vi "QMH_Demo_1.vi"(11 "Sender":string="Demo_1") -> ()   [LabVIEW 2014]
panel:
  in  "Receiver":string="Demo"
  out "Receive data":string
  in  "Send data":string
  in  "STOP":bool
  in  "send":bool
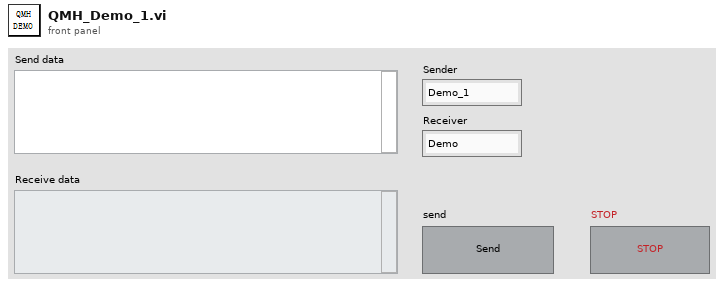
[diagram p1: front panel]
types:
  T1 = cluster{"Communication message":cluster{"Sender":string, "receiver":string, "message":string, "data":variant}, "Receive data":string}
  T2 = cluster{"Sender":string, "receiver":string, "message":string, "data":variant}
  T3 = enum32{"invalid app kind", "Development System", "Run Time System", "Student Edition", "Embedded LabVIEW", "Evaluation", "Custom"}
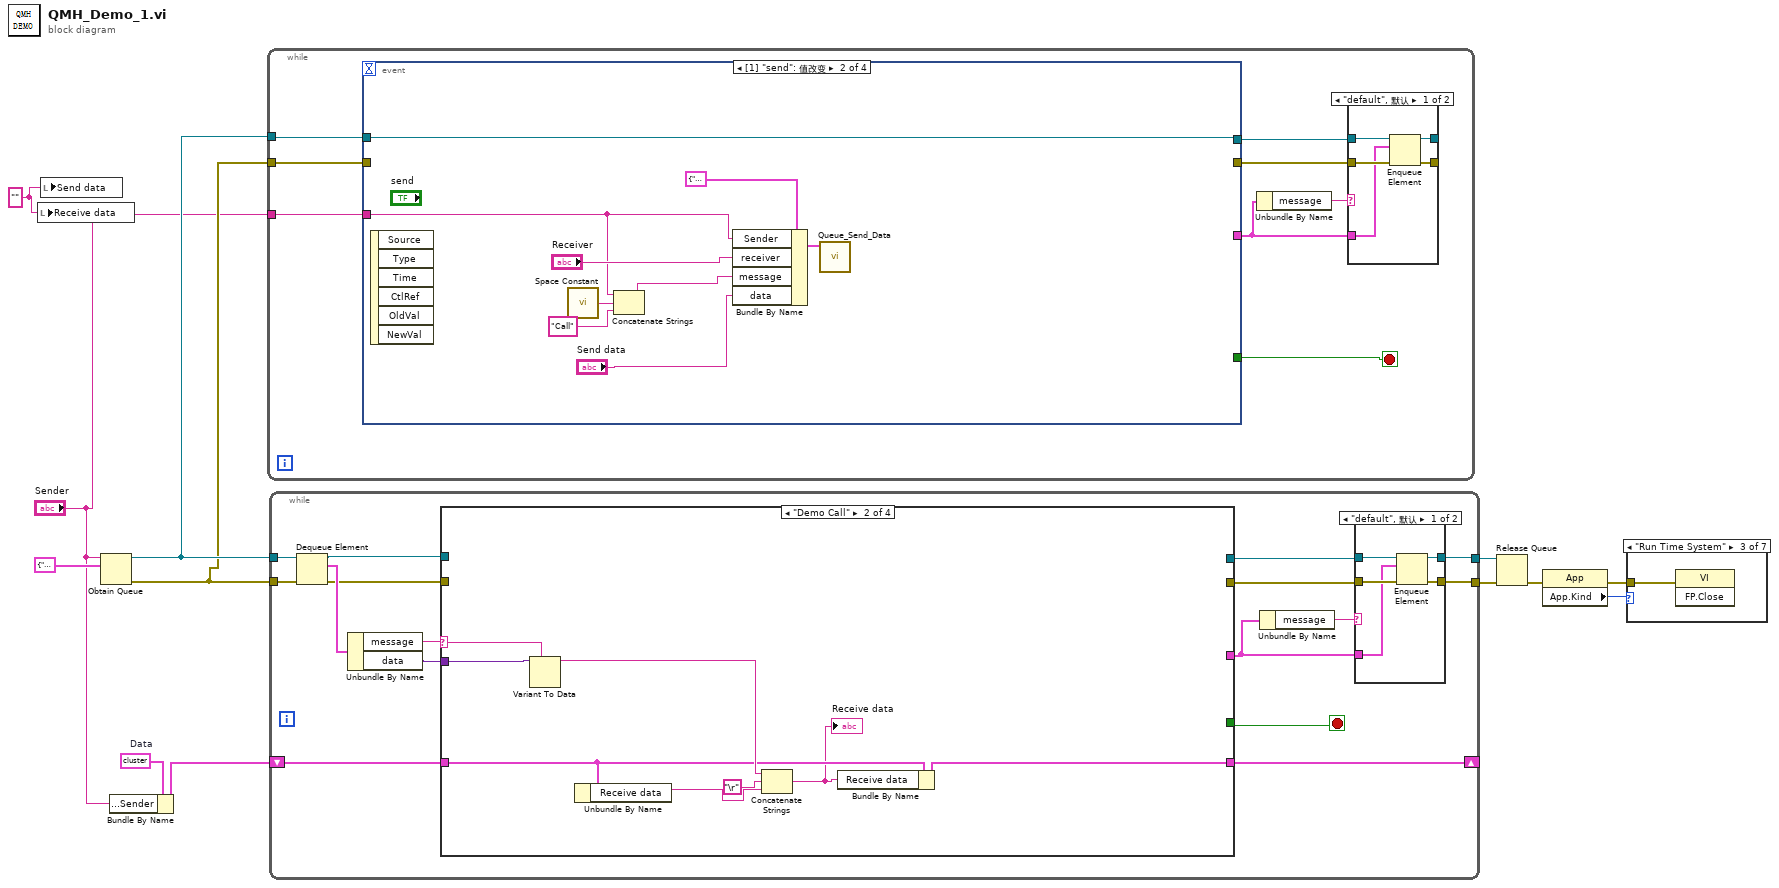
[diagram p0: block diagram]
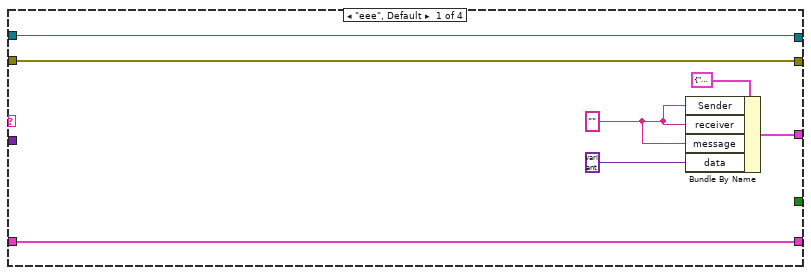
[diagram p9: hidden frame]
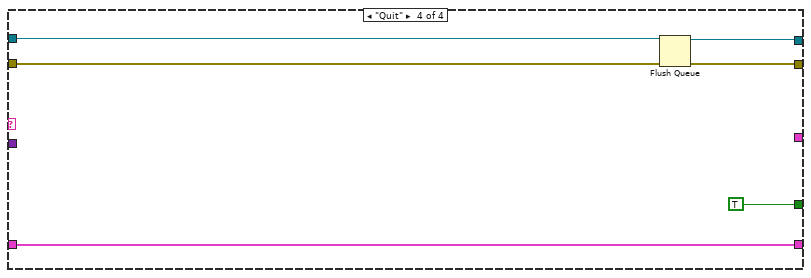
[diagram p11: hidden frame]
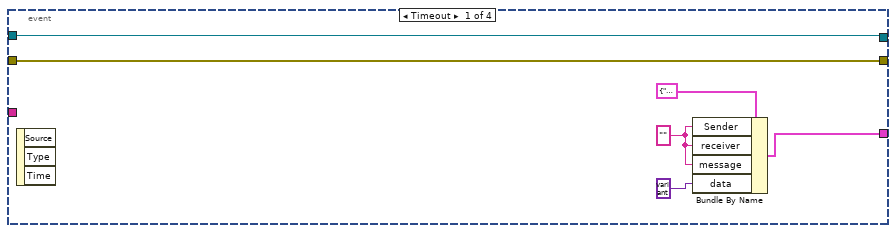
[diagram p13: hidden frame]
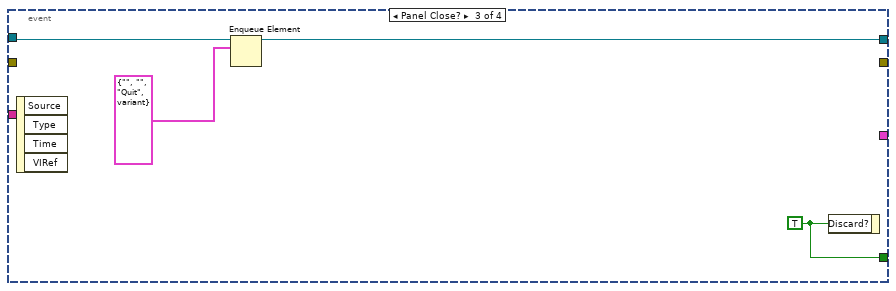
[diagram p14: hidden frame]
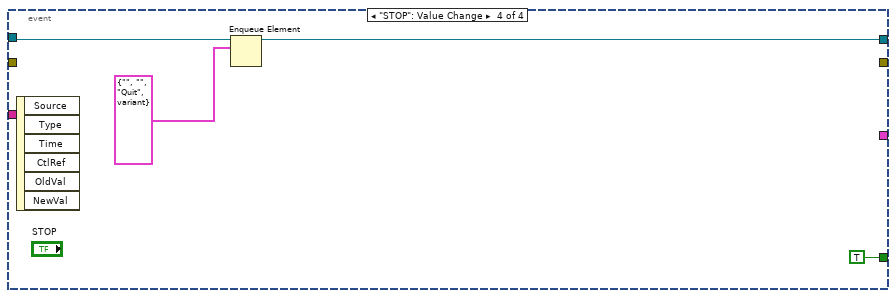
[diagram p15: hidden frame]
diagram:
  w1 = "" ("message")
  w4 = T1 {"Communication message"={"Sender"="", "receiver"="", "message"="", "data"=variant}, "Receive data"=""}  # Data
  n1 = local write "Receive data"(w1) -> ()
  n2 = local write "Send data"(w1) -> ()
  n3 = Obtain Queue(name (unnamed)="Sender", element data type=T2 {"Sender"="", "receiver"="", "message"="", "data"=variant} ("Communication message")) -> (queue out=w12:refnum<queue>, error out=w5:errorcluster)  [unwired: 3 in, 1 out]
  n4 = Bundle By Name(cluster=w4, "Communication message.Sender"="Sender") -> (w3:T1)
  n5 = while {
    tunnel: w12 -> [w19]
    tunnel: w5 -> [w17]
    tunnel: "Sender" -> [w13]
    stop <- w20 stop-if-true
    n6 = event shown="[1] \"send\": 值改变" {
      selector: _ -> [_ _ _ _]
      dyn-events: _ -> [_ _ _ _]
      timeout: _ -> [_ _ _ _]
      tunnel: [_ _ w46 TRUE ("放弃？")] -> w20
      tunnel: w19 -> [w30 w42 w45 w49]
      tunnel: [w30 w42 w43 w47] -> w18
      tunnel: [w32 _ _ _] -> w15
      tunnel: [w29 _ _ _] -> w16
      tunnel: w17 -> [w29 _ _ _]
      tunnel: w13 -> [_ w36 _ _]
      event Timeout {
        w28 = ""
        n7 = event-data() -> ()  [unwired: 1 in, 3 out]
        n8 = Bundle By Name(cluster=T2 {"Sender"="", "receiver"="", "message"="", "data"=variant} ("Communication message"), "Sender"=w28, "receiver"=w28, "message"=w28, "data"=variant) -> (w32:T2)
      }
      event "send": Value Change {
        n9 = event-data() -> ()  [unwired: 1 in, 6 out]
        n10 = call <vilib>:"Space Constant.vi"() -> ("String"=w35:string)
        n11 = Concatenate Strings(w36, w35, "Call" ("message")) -> (w37:string)
        n12 = Bundle By Name(cluster=T2 {"Sender"="", "receiver"="", "message"="", "data"=variant} ("Communication message"), "Sender"=w36, "receiver"="Receiver", "message"=w37, "data"="Send data") -> (w40:T2)
        n13 = call "Queue_Send_Data.vi"("Communication message"=w40) -> ()  [unwired: 10 in, 1 out]
      }
      event Panel Close? {
        w46 = TRUE ("放弃？")
        n14 = event-data() -> ()  [unwired: 1 in, 4 out]
        n15 = Enqueue Element(queue=w45, element=T2 {"Sender"="", "receiver"="", "message"="Quit", "data"=variant} ("Communication message")) -> (queue out=w43:refnum<queue>)  [unwired: 2 in, 2 out]
        n16 = event-data("Discard?"=w46) -> ()  [unwired: 1 in, 1 out]
      }
      event "STOP": Value Change {
        n17 = event-data() -> ()  [unwired: 1 in, 6 out]
        n18 = Enqueue Element(queue=w49, element=T2 {"Sender"="", "receiver"="", "message"="Quit", "data"=variant} ("Communication message")) -> (queue out=w47:refnum<queue>)  [unwired: 2 in, 2 out]
      }
    }
    n19 = Unbundle By Name(w15) -> ("message"=w14:string)
    n20 = case shown="\"default\", 默认" w14 {
      tunnel: w18 -> [w25 w27]
      tunnel: w16 -> [w24 w26]
      tunnel: w15 -> [w23 _]
      tunnel: [w22 w27] -> _
      tunnel: [w21 w26] -> _
      frame "default", Default {
        n21 = Enqueue Element(queue=w25, element=w23, error in (no error)=w24) -> (queue out=w22:refnum<queue>, error out=w21:errorcluster)  [unwired: 1 in, 1 out]
      }
      frame "" {
      }
    }
  }
  n22 = while {
    tunnel: w12 -> [w66]
    tunnel: w5 -> [w65]
    tunnel: [w57] -> w11
    tunnel: [w56] -> w10
    shift-right: [w51] -> _
    shift-left: w3 -> [w52]
    stop <- w55 stop-if-true
    n23 = Dequeue Element(queue=w66, error in (no error)=w65) -> (queue out=w62:refnum<queue>, element=w64:T2, error out=w61:errorcluster)  [unwired: 1 in, 1 out]
    n24 = Unbundle By Name(w64) -> ("message"=w63:string, "data"=w58:variant)
    n25 = case shown="\"Demo Call\"" w63 {
      selector: w63 -> [_ w87 _ _]
      tunnel: [w80 _ w91 w96] -> w60
      tunnel: w62 -> [w80 _ w91 w95]
      tunnel: w61 -> [w79 _ w90 w93]
      tunnel: [w79 _ w90 w94] -> w59
      tunnel: w58 -> [_ w88 _ _]
      tunnel: [_ _ _ TRUE] -> w55
      tunnel: [w77 _ _ _] -> w54
      tunnel: [w74 w82 w89 w92] -> w51
      tunnel: w52 -> [w74 w84 w89 w92]
      frame "eee", Default {
        w75 = ""
        n26 = Bundle By Name(cluster=T2 {"Sender"="", "receiver"="", "message"="", "data"=variant} ("Communication message"), "Sender"=w75, "receiver"=w75, "message"=w75, "data"=variant) -> (w77:T2)
      }
      frame "Demo Call" {
        n27 = Variant To Data(type=w87, Variant=w88) -> (data=w86:string)  [unwired: 1 in, 1 out]
        n28 = Unbundle By Name(w84) -> ("Receive data"=w83:string)
        n29 = Concatenate Strings(w86, "\r", w83) -> (w81:string)
        "Receive data" <- w81
        n30 = Bundle By Name(cluster=w84, "Receive data"=w81) -> (w82:T1)
      }
      frame "Init" {
      }
      frame "Quit" {
        n31 = Flush Queue(queue=w95, error in (no error)=w93) -> (queue out=w96:refnum<queue>, error out=w94:errorcluster)  [unwired: 1 out]
      }
    }
    n32 = Unbundle By Name(w54) -> ("message"=w53:string)
    n33 = case shown="\"default\", 默认" w53 {
      tunnel: w60 -> [w71 w73]
      tunnel: w59 -> [w70 w72]
      tunnel: w54 -> [w69 _]
      tunnel: [w68 w73] -> w57
      tunnel: [w67 w72] -> w56
      frame "default", Default {
        n34 = Enqueue Element(queue=w71, element=w69, error in (no error)=w70) -> (queue out=w68:refnum<queue>, error out=w67:errorcluster)  [unwired: 1 in, 1 out]
      }
      frame "" {
      }
    }
  }
  n35 = Release Queue(queue=w11, error in (no error)=w10) -> (error out=w9:errorcluster)  [unwired: 1 in, 2 out]
  n36 = property class="App"(error in=w9) -> (error out=w8:errorcluster, "App.Kind"=w7:T3)  [unwired: 1 in, 1 out]
  n37 = case shown="\"Run Time System\"" w7 {
    tunnel: w8 -> [_ _ w98 _ _ _ _]
    frame "invalid app kind", Default {
    }
    frame "Development System" {
    }
    frame "Run Time System" {
      n38 = invoke class="VI" method="FP.Close"(error in=w98) -> ()  [unwired: 2 in, 3 out]
    }
    frame "Student Edition" {
    }
    frame "Embedded LabVIEW" {
    }
    frame "Evaluation" {
    }
    frame "Custom" {
    }
  }
